vi "VI Fitxers.vi"(6 "Array in":u32[](array[numeric]), 9 "access (0:read/write)":enum16{"read/write", "read-only", "write-only"}(ring), 10 "operation (0:open)":T1(ring), 11 "file path (use dialog)":path) -> (0 "error out":errorcluster)   [LabVIEW 2017]
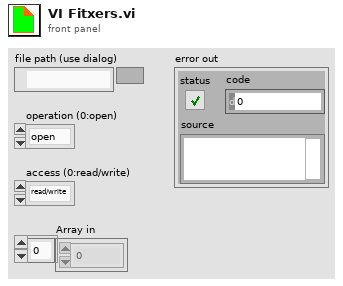
[diagram p1: front panel]
types:
  T1 = enum16{"open", "replace", "create", "open or create", "replace or create", "replace or create with confirmation"}
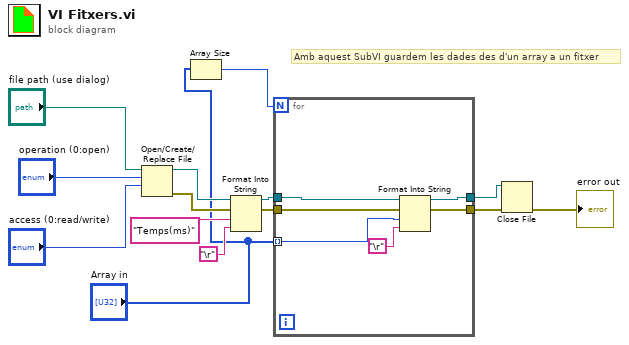
[diagram p0: block diagram]
diagram:
  # "Amb aquest SubVI guardem les dades des d'un array a un fitxer"
  n1 = Open/Create/Replace File(file path (use dialog)="file path (use dialog)", operation (0:open)="operation (0:open)", access (0:read/write)="access (0:read/write)") -> (refnum out=w9:refnum<file>, error out=w10:errorcluster)  [unwired: 3 in, 1 out]
  n2 = Array Size(array="Array in") -> (size(s)=w14:i32)
  n3 = Format Into String(initial string=w9, error in=w10, "Temps(ms)", "\r") -> (resulting string=w11:refnum<file>, error out=w12:errorcluster)  [unwired: 1 in]
  n4 = for {
    N: w14 -> [_]
    tunnel: w11 -> [w20]
    tunnel: [w19] -> w5
    tunnel: [w18] -> w6
    tunnel: w12 -> [w17]
    tunnel: "Array in" -> [w15] mode=indexing
    n5 = Format Into String(initial string=w20, error in=w17, w15, "\r") -> (resulting string=w19:refnum<file>, error out=w18:errorcluster)  [unwired: 1 in]
  }
  n6 = Close File(refnum=w5, error in=w6) -> (error out=→"error out":errorcluster)  [unwired: 1 out]
